vi "Voltage2Current.vi"(0 "电流值":dbl, 5 "校准矩阵":sgl[][](array[numeric])) -> (6 "偏压(V)":dbl, 8 "VI量程":bool[](array[boolean]))   [LabVIEW 2020]
doc: "I. Description:\nThis example demonstrates how to acquire a continuous amount of data (Waveform) using the DAQ device's internal clock.\n\nII. Instructions for Running:\n1. Select the physical channel to correspond to where your signal is input on the DAQ device.\n2. Enter the minimum and maximum voltages.\nNote: For better accuracy try to match the input range to the expected voltage level of the measured signal.\n3. Select the number of samples to acquire per loop iteration.\n4. Set the rate of the acquisition\nNote: The rate should be AT LEAST twice as fast as the maximum frequency component of the signal being acquired.\n\nIII. Block Diagram Steps:\n1. Create an analog input voltage channel.\n2. Set the rate for the sample clock. Additionally, define the sample mode to be continuous.\n3. Call the Start VI to start the acquisition.\n4. Read the waveform data in a loop until the user hits the stop button or an error occurs.\nNote: This example reads data from one or more channels and returns an array of data. Use the Index Array function to access an individual channel of data.\n5. Call the Clear Task VI to clear the Task.\n6. Use the popup dialog box to display an error if any.\n\nIV. I/O Connections Overview:\nMake sure your signal input terminal matches the Physical Channel I/O Control. For further connection information, refer to your hardware reference manual."
uses:
  <vilib>/Analysis/polynomials.llb/Scalar Polynomial Evaluation (DBL).vi
  <vilib>/Analysis/NI_AALPro.lvlib
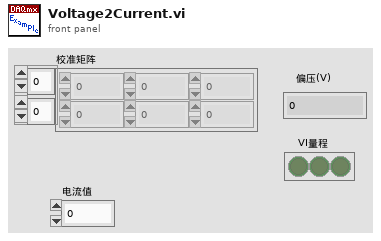
[diagram p1: front panel]
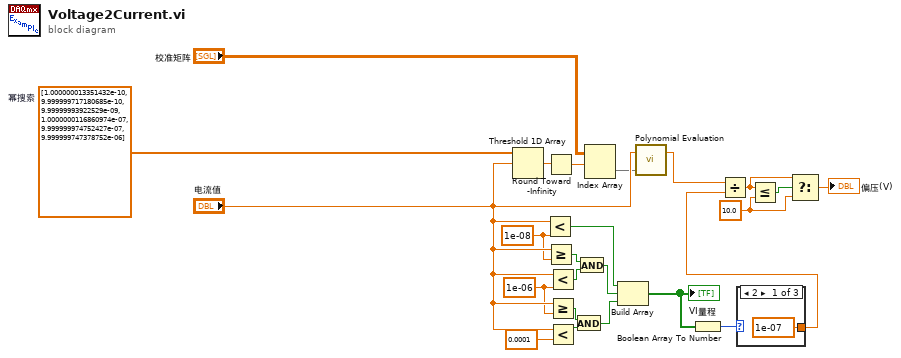
[diagram p0: block diagram]
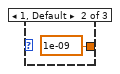
[diagram p2: hidden frame]
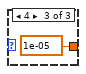
[diagram p3: hidden frame]
diagram:
  w2 = 10.0 ("y")
  w17 = 1e-06 ("y")
  w20 = 1e-08 ("y")
  w24 = sgl[] [1e-10, 1e-09, 1e-08, 1e-07, 1e-06, 1e-05]  # 幂搜索
  n1 = Threshold 1D Array(2:"电流值", 3:w24) -> (0:w9:sgl)  [unwired: 1 in]
  n2 = Less?(x="电流值", y=w20) -> (x < y?=w13:bool)
  n3 = Round Toward -Infinity ("向下取整")(1:w9) -> (0:w8:sgl)
  n4 = Greater Or Equal?(x="电流值", y=w20) -> (x >= y?=w18:bool)
  n5 = Less?(x="电流值", y=w17) -> (x < y?=w19:bool)
  n6 = Greater Or Equal?(x="电流值", y=w17) -> (x >= y?=w16:bool)
  n7 = Less?(x="电流值", y=0.0001) -> (x < y?=w15:bool)
  n8 = And(x=w16, y=w15) -> (x .and. y?=w11:bool)
  n9 = And(x=w18, y=w19) -> (x .and. y?=w12:bool)
  n10 = Index Array(array="校准矩阵", index (row)=w8) -> (element=w7:sgl[])  [unwired: 1 in]
  n11 = Build Array(w13, w12, w11) -> (w5:bool[])
  "VI量程" <- w5
  n12 = call-poly <vilib>:"Polynomial Evaluation.vi"("P(x)"=w7, "a"="电流值") -> ("P(a)"=w6:dbl)  [unwired: 1 out]
  n13 = Boolean Array To Number(Boolean array=w5) -> (number=w21:u32)
  n14 = case shown="2" w21 {
    tunnel: [1e-07 ("timeout") 1e-09 ("timeout") 1e-05 ("timeout")] -> w10
    frame 2 {
    }
    frame 1, Default {
    }
    frame 4 {
    }
  }
  n15 = Divide(x=w6, y=w10) -> (x/y=w3:dbl)
  n16 = Less Or Equal?(x=w3, y=w2) -> (x <= y?=w4:bool)
  n17 = Select(t=w3, s=w4, f=w2) -> (s? t:f=→"偏压(V)":dbl)
